vi "Autonomous_Globals.vi"() -> ()   [LabVIEW 2020]
panel:
  out "Autonomous_Play_Done":bool
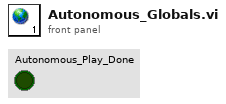
[diagram p1: front panel]
diagram:
